vi "readSetting.vi"(8 "error in (no error)":errorcluster, 10 "Path":path=path "/home/ttsai/Documents/stash/ts_tcs_ofc/configData/pinv.esti", 11 "OptStateEsti in":refnum<class "OptStateEsti.lvclass">) -> (0 "error out":errorcluster, 3 "OptStateEsti out":refnum<class "OptStateEsti.lvclass">)   [LabVIEW 2016, in "OptStateEsti.lvclass"]
doc: "Read the configuration setting file of optical state estimator."
uses:
  OptStateEsti.lvclass
  OptStateEsti.lvclass/OptStateEsti.ctl
panel:
  in  "Parameter List":string[](array[string])=["estimator_strategy", "znmax", "izn3", "icomp"]
  in  "Array Parameter List":string[](array[string])=["izn3", "icomp"]
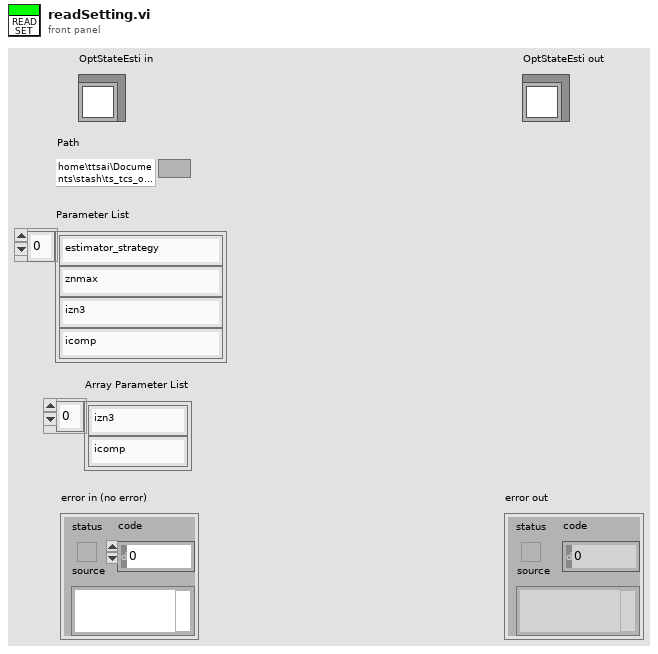
[diagram p1: front panel]
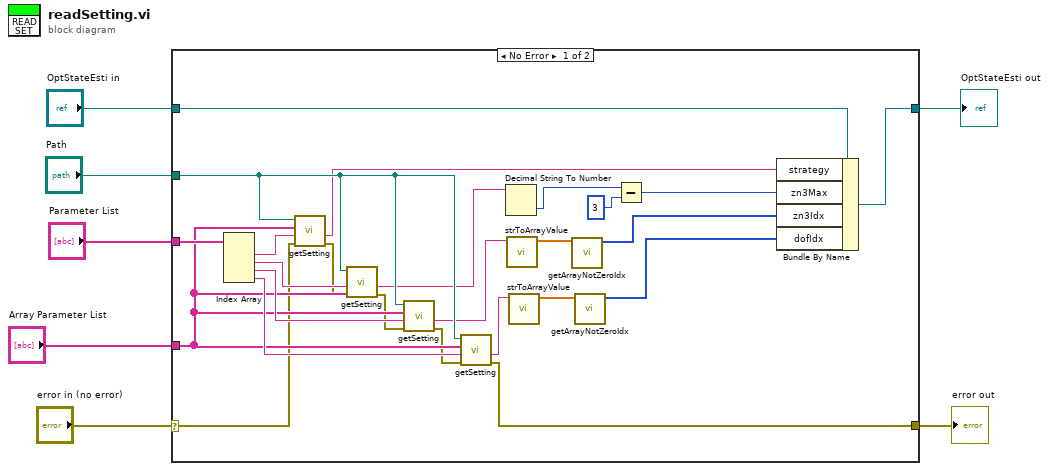
[diagram p0: block diagram]
diagram:
  n1 = case shown="No Error" "error in (no error)" {
    selector: "error in (no error)" -> [w25 w34]
    tunnel: [w21 w34] -> w6
    tunnel: [w19 w33] -> w4
    tunnel: "OptStateEsti in" -> [w20 w33]
    tunnel: "Path" -> [w30 _]
    tunnel: "Array Parameter List" -> [w26 _]
    tunnel: "Parameter List" -> [w32 _]
    frame No Error {
      n2 = Index Array(array=w32) -> (element #1=w31:string, element #2=w29:string, element #3=w28:string, element #4=w27:string)  [unwired: 4 in]
      n3 = call "getSetting.vi"("error in"=w25, "Parameter"=w31, "Array Parameter List"=w26, "Path"=w30) -> ("error out"=w24:errorcluster, "Value"=w18:string)  [unwired: 6 in]
      n4 = call "getSetting.vi"("error in"=w24, "Parameter"=w29, "Array Parameter List"=w26, "Path"=w30) -> ("error out"=w23:errorcluster, "Value"=w17:string)  [unwired: 6 in]
      n5 = call "getSetting.vi"("error in"=w23, "Parameter"=w28, "Array Parameter List"=w26, "Path"=w30) -> ("error out"=w22:errorcluster, "Value"=w16:string)  [unwired: 6 in]
      n6 = call "getSetting.vi"("error in"=w22, "Parameter"=w27, "Array Parameter List"=w26, "Path"=w30) -> ("error out"=w21:errorcluster, "Value"=w15:string)  [unwired: 6 in]
      n7 = Decimal String To Number(string=w17) -> (number=w14:i32)  [unwired: 2 in, 1 out]
      n8 = call "strToArrayValue.vi"("String"=w16) -> ("Array"=w10:dbl[])  [unwired: 10 in]
      n9 = call "strToArrayValue.vi"("String"=w15) -> ("Array"=w11:dbl[])  [unwired: 10 in]
      n10 = call "getArrayNotZeroIdx.vi"("Array"=w10) -> ("Index Array"=w9:i32[])  [unwired: 10 in]
      n11 = call "getArrayNotZeroIdx.vi"("Array"=w11) -> ("Index Array"=w8:i32[])  [unwired: 10 in]
      n12 = Subtract(x=w14, y=3) -> (x-y=w12:i32)
      n13 = Bundle By Name(cluster=w20, "strategy"=w18, "zn3Max"=w12, "zn3Idx"=w9, "dofIdx"=w8) -> (w19:refnum<class "OptStateEsti.lvclass">)
    }
    frame Error {
    }
  }
  "error out" <- w6
  "OptStateEsti out" <- w4
